vi "Get Class Functions C Description.vi"(8 "error in (no error)":errorcluster, 10 "Access Scope":T1(ring)=enum."public", 11 "LabVIEW Obj":refnum<class>) -> (0 "error out":errorcluster, 3 "Array":string[](array[string]))   [LabVIEW 2017]
uses:
  <userlib>/_OpenG.lib/string/string.llb/Trim Whitespace (String)__ogtk.vi
  <vilib>/Utility/VariantDataType/VariantType.lvlib
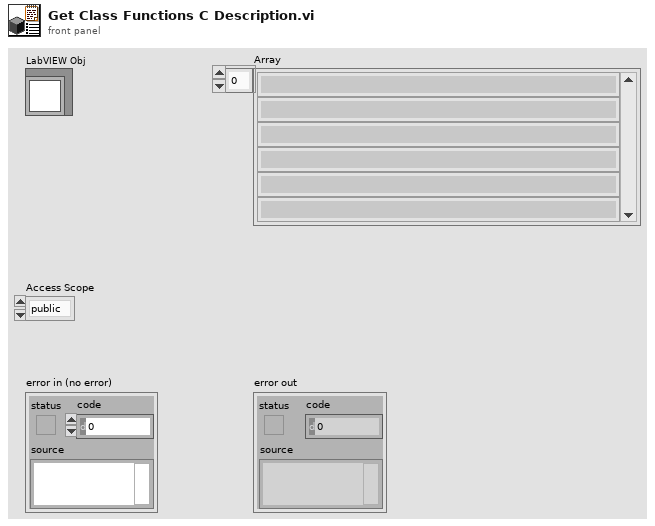
[diagram p1: front panel]
types:
  T1 = enum32{"invalid scope", "public", "private", "protected", "community"}
  T2 = typedef "VariantType.lvlib/VIInfo.ctl" = cluster{"Data1":i16, "Data2":i16, "Flags":u32[], "Modification Date":timestamp, "Asynchronous":bool, "NonFunctional":bool, "Subroutine":bool, "SubSystem":bool}
  T3 = typedef "Type Descriptor Enumeration__ogtk.ctl" = enum8{"<Null>", "I8", "I16", "I32", "I64", "U8", "U16", "U32", "U64", "SGL", "DBL", "EXT", "CSG", "CDB", "CXT", "0x0F", "0x10", "0x11", "0x12", "0x13", "0x14", "Enum U8", "Enum U16", "Enum U32", "Enum U64", "SGL PQ", "DBL PQ", "EXT PQ", "CSG PQ", "CDB PQ", "CXT PQ", "0x1F", "0x20", "Boolean", "0x22", "0x23", "0x24", "0x25", "0x26", "0x27", "0x28", "0x29", "0x2A", "0x2B", "0x2C", "0x2D", "0x2E", "0x2F", "String", "0x31", "Path", "Pict", "0x34", "0x35", "0x36", "DAQ", "0x38", "0x39", "0x3A", "0x3B", "0x3C", "0x3D", "0x3E", "0x3F", "Array", "0x41", "0x42", "0x43", "0x44", "0x45", "0x46", "0x47", "0x48", "0x49", "0x4A", "0x4B", "0x4C", "0x4D", "0x4E", "0x4F", "Cluster", "0x51", "0x52", "Variant", "Waveform", "0x55", "0x56", "0x57", "0x58", "0x59", "0x5A", "0x5B", "0x5C", "0x5D", "0x5E", "0x5F", "0x60", "0x61", "0x62", "0x63", "0x64", "0x65", "0x66", "0x67", "0x68", "0x69", "0x6A", "0x6B", "0x6C", "0x6D", "0x6E", "0x6F", "Refnum"}
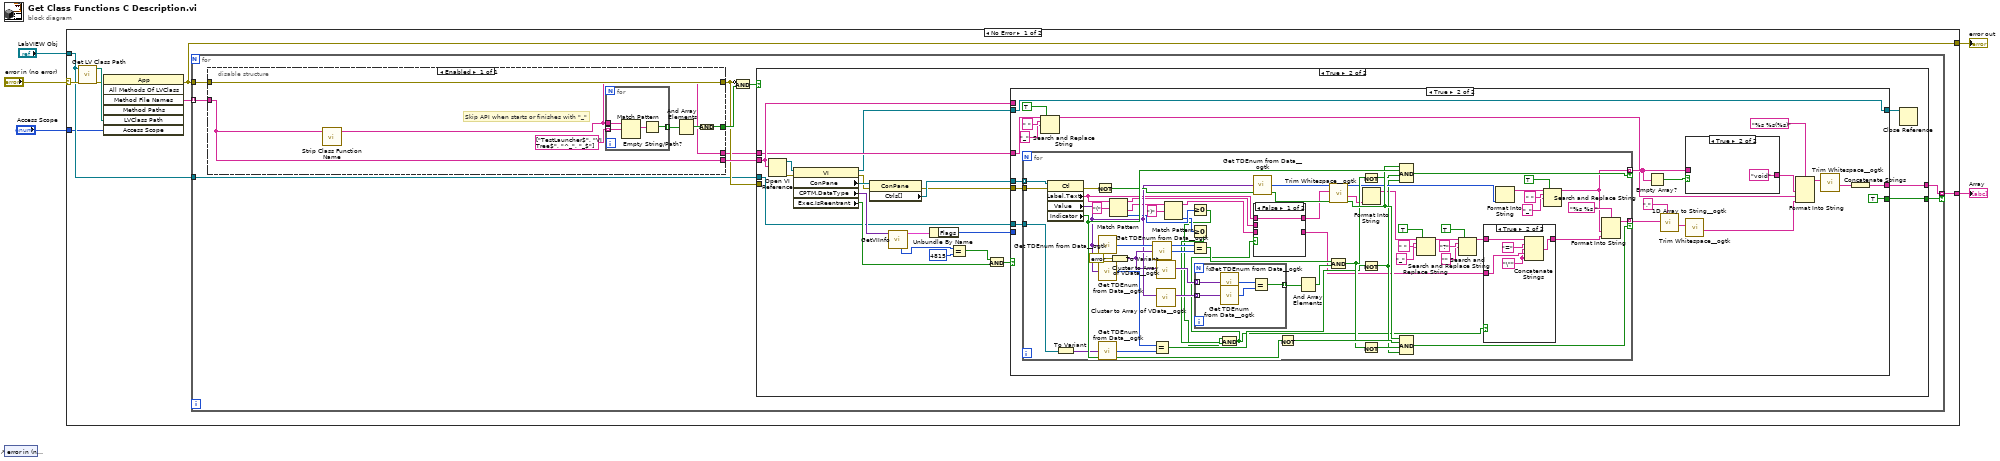
[diagram p0: block diagram]
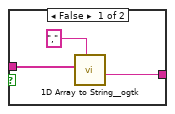
[diagram p4: hidden frame]
diagram:
  n1 = control-ref of="error in (no error)"() -> ()  [unwired: 1 out]
  n2 = case shown="No Error" "error in (no error)" {
    selector: "error in (no error)" -> [w12 w155]
    tunnel: [w9 w155] -> w4
    tunnel: "LabVIEW Obj" -> [w7 _]
    tunnel: [w8 _] -> w2
    tunnel: "Access Scope" -> [w6 _]
    frame No Error {
      n3 = call <vilib>:"Get LV Class Path.vi"("error in (no error)"=w12, "object"=w7) -> ("error out"=w10:errorcluster, "class path"=w13:path)  [unwired: 8 in]
      n4 = invoke class="App" method="All Methods Of LVClass"(error in=w10, "LVClass Path"=w13, "Access Scope"=w6) -> (error out=w9:errorcluster, "Method File Names"=w11:string[])  [unwired: 4 in, 5 out]
      n5 = for {
        tunnel: w11 -> [w19] mode=indexing
        tunnel: [w23] -> w8 mode=indexing if=w22
        tunnel: w9 -> [w20]
        tunnel: w7 -> [w14]
        n6 = disable-structure shown="Enabled" {
          disable-tunnel: [w24] -> w21
          disable-tunnel: w20 -> [w27]
          disable-tunnel: w19 -> [w24]
          disable-tunnel: [w26] -> w18
          disable-tunnel: [w27] -> w16
          disable-tunnel: [w25] -> w15
          frame Enabled {
            # "Skip API when starts or finishes with \"_\""
            n7 = call "Strip Class Function Name.vi"("File Full Path Name"=w24) -> ("Function Name"=w25:string)  [unwired: 2 in, 2 out]
            n8 = for {
              tunnel: w25 -> [w34]
              tunnel: string[] ["TestLauncher$", "VI Tree$", "^_", "_$"] -> [w33] mode=indexing
              tunnel: [w31] -> w28 mode=indexing
              n9 = Match Pattern(string=w34, regular expression=w33) -> (match substring=w32:string)  [unwired: 1 in, 3 out]
              n10 = Empty String/Path?(string/path=w32) -> (empty?=w31:bool)
            }
            n11 = And Array Elements(Boolean array=w28) -> (logical AND=w30:bool)
            n12 = Compound Arithmetic op=AND(w30) -> (w26:bool)
          }
        }
        n13 = Compound Arithmetic op=AND(invert w16, w18) -> (w17:bool)
        n14 = case shown="True" w17 {
          tunnel: [_ w55] -> w23
          tunnel: [_ w54] -> w22
          tunnel: w21 -> [_ w53]
          tunnel: w16 -> [_ _]
          tunnel: w15 -> [_ w52]
          tunnel: w14 -> [_ w35]
          frame False {
          }
          frame True {
            n15 = Open VI Reference(vi path=w53) -> (vi reference=w47:refnum<vi>, error out=w48:errorcluster)  [unwired: 5 in]
            n16 = property class="VI"(reference=w47, error in=w48) -> (reference out=w38:refnum<vi>, error out=w46:errorcluster, "ConPane"=w51:refnum<vi>, "CPTM.DataType"=w45:variant, "Exec.IsReentrant"=w39:bool)
            n17 = property class="ConPane"(reference=w51, error in=w46) -> (error out=w36:errorcluster, "Ctrls[]"=w50:refnum<vi>[])  [unwired: 1 out]
            n18 = call <vilib>:"GetVIInfo.vi"("Variant"=w45) -> ("VI Info"=w43:T2, "pattern"=w44:i16)  [unwired: 6 in, 3 out]
            n19 = Unbundle By Name(w43) -> ("Flags"=w42:u32[])
            n20 = Equal?(x=w44, y=i16 4815) -> (x = y?=w41:bool)
            n21 = Compound Arithmetic op=AND(w41, w39) -> (w40:bool)
            n22 = case shown="True" w40 {
              tunnel: [_ w57] -> w55
              tunnel: w50 -> [_ w76]
              tunnel: [_ TRUE] -> w54
              tunnel: w53 -> [_ _]
              tunnel: w52 -> [_ w61]
              tunnel: w42 -> [_ _]
              tunnel: w38 -> [w56 w77]
              tunnel: [w56 w77] -> w37
              tunnel: w36 -> [_ w69]
              tunnel: w35 -> [_ w67]
              frame False {
              }
              frame True {
                n23 = for {
                  tunnel: w76 -> [w140] mode=indexing
                  tunnel: [w102] -> w66 mode=indexing if=w133
                  tunnel: [w138] -> w74 mode=indexing if=w132
                  tunnel: w69 -> [w135]
                  tunnel: w67 -> [w116]
                  n24 = property class="Ctl"(reference=w140, error in=w135) -> (error out=w134:errorcluster, "Label.Text"=w95:string, "Value"=w115:variant, "Indicator"=w137:bool)  [unwired: 1 out]
                  n25 = To Variant(anything=w116) -> (Variant=w117:variant)
                  n26 = Not(x=w134) -> (.not. x?=w131:bool)
                  n27 = call <userlib>:"Get TDEnum from Data__ogtk.vi"("Data"=w115) -> ("Type Descriptor Enumeration"=w129:T3)  [unwired: 4 in]
                  n28 = call <userlib>:"Get TDEnum from Data__ogtk.vi"("Data"=w115) -> ("Type Descriptor Enumeration"=w114:T3)  [unwired: 4 in]
                  n29 = call <userlib>:"Get TDEnum from Data__ogtk.vi"("Data"=w117) -> ("Type Descriptor Enumeration"=w113:T3)  [unwired: 4 in]
                  n30 = Match Pattern(string=w95, regular expression="(") -> (before substring=w93:string, after substring=w88:string, offset past match=w99:i32)  [unwired: 1 in, 1 out]
                  n31 = To Variant(anything=errorcluster {"status"=FALSE, "code"=0, "source"=""} ("error in (no error)")) -> (Variant=w127:variant)
                  n32 = call <userlib>:"Get TDEnum from Data__ogtk.vi"("Data"=w127) -> ("Type Descriptor Enumeration"=w128:T3)  [unwired: 4 in]
                  n33 = Equal?(x=w114, y=w113) -> (x = y?=w112:bool)
                  n34 = call <userlib>:"Cluster to Array of VData__ogtk.vi"("Cluster"=w127) -> ("Array of VData"=w126:variant[])  [unwired: 9 in, 1 out]
                  n35 = call <userlib>:"Cluster to Array of VData__ogtk.vi"("Cluster"=w115) -> ("Array of VData"=w125:variant[])  [unwired: 9 in, 1 out]
                  n36 = Match Pattern(string=w88, regular expression=")") -> (before substring=w89:string, offset past match=w98:i32)  [unwired: 1 in, 2 out]
                  n37 = Greater Or Equal To 0?(x=w99) -> (x >= 0?=w96:bool)
                  n38 = Greater Or Equal To 0?(x=w98) -> (x >= 0?=w97:bool)
                  n39 = Equal?(x=w129, y=w128) -> (x = y?=w124:bool)
                  n40 = for {
                    tunnel: w126 -> [w154] mode=indexing
                    tunnel: w125 -> [w153] mode=indexing
                    tunnel: [w150] -> w123 mode=indexing
                    n41 = call <userlib>:"Get TDEnum from Data__ogtk.vi"("Data"=w154) -> ("Type Descriptor Enumeration"=w152:T3)  [unwired: 4 in]
                    n42 = call <userlib>:"Get TDEnum from Data__ogtk.vi"("Data"=w153) -> ("Type Descriptor Enumeration"=w151:T3)  [unwired: 4 in]
                    n43 = Equal?(x=w152, y=w151) -> (x = y?=w150:bool)
                  }
                  n44 = And(x=w96, y=w97) -> (x .and. y?=w92:bool)
                  n45 = call <userlib>:"Get TDEnum from Data__ogtk.vi"("Data"=w115) -> ("Type Descriptor Enumeration"=w118:T3)  [unwired: 4 in]
                  n46 = case shown="False" w92 {
                    tunnel: [w147 w149] -> w94
                    tunnel: w95 -> [w147 _]
                    tunnel: w93 -> [_ w149]
                    tunnel: [_ w148] -> w90
                    tunnel: w89 -> [_ w148]
                    frame False {
                    }
                    frame True {
                    }
                  }
                  n47 = Not(x=w137) -> (.not. x?=w136:bool)
                  n48 = And Array Elements(Boolean array=w123) -> (logical AND=w121:bool)
                  n49 = call-poly <userlib>:"Trim Whitespace__ogtk.vi"("String in"=w94) -> ("String out"=w87:string)  [unwired: 6 in]
                  n50 = Compound Arithmetic op=AND(w124, w121) -> (w122:bool)
                  n51 = Not(x=w122) -> (.not. x?=w119:bool)
                  n52 = Not(x=w122) -> (.not. x?=w120:bool)
                  n53 = Format Into String(w87) -> (resulting string=w103:string)  [unwired: 3 in, 1 out]
                  n54 = Not(x=w112) -> (.not. x?=w111:bool)
                  n55 = Compound Arithmetic op=AND(w131, w137, w119, w111) -> (w133:bool)
                  n56 = Compound Arithmetic op=AND(w131, w136, w120, w111) -> (w132:bool)
                  n57 = Search and Replace String(replace all?=TRUE ("replace all? (F)"), input string=w103, search string=" ", replace string="_" ("replace string (\"\")")) -> (result string=w83:string)  [unwired: 4 in, 3 out]
                  n58 = Search and Replace String(replace all?=TRUE ("replace all? (F)"), input string=w83, search string="?", replace string="" ("replace string (\"\")")) -> (result string=w82:string)  [unwired: 4 in, 3 out]
                  n59 = case shown="True" w92 {
                    tunnel: w82 -> [w141 w145]
                    tunnel: [w141 w146] -> w91
                    tunnel: w90 -> [_ w143]
                    frame False {
                    }
                    frame True {
                      w142 = "\"" ("string")
                      n60 = Concatenate Strings(w145, "=" ("string"), w142, w143, w142) -> (w146:string)
                    }
                  }
                  n61 = Format Into String(w118) -> (resulting string=w110:string)  [unwired: 3 in, 1 out]
                  n62 = Search and Replace String(replace all?=TRUE ("replace all? (F)"), input string=w110, search string=" ", replace string="_" ("replace string (\"\")")) -> (result string=w102:string)  [unwired: 4 in, 3 out]
                  n63 = Format Into String(format string="%s %s ", w102, w91) -> (resulting string=w138:string)  [unwired: 2 in, 1 out]
                }
                n64 = Search and Replace String(replace all?=TRUE ("replace all? (F)"), input string=w61, search string=" ", replace string="_" ("replace string (\"\")")) -> (result string=w60:string)  [unwired: 4 in, 3 out]
                n65 = Empty Array?(array=w66) -> (empty?=w65:bool)
                n66 = call <userlib>:"1D Array to String__ogtk.vi"("delimiter (Tab)"=",", "Array of Strings"=w74) -> ("delimited string"=w71:string)  [unwired: 9 in]
                n67 = case shown="True" w65 {
                  tunnel: [w79 "void" ("delimited string")] -> w72
                  tunnel: w66 -> [w78 _]
                  frame False {
                    n68 = call <userlib>:"1D Array to String__ogtk.vi"("delimiter (Tab)"=",", "Array of Strings"=w78) -> ("delimited string"=w79:string)  [unwired: 9 in]
                  }
                  frame True {
                  }
                }
                n69 = call-poly <userlib>:"Trim Whitespace__ogtk.vi"("String in"=w71) -> ("String out"=w58:string)  [unwired: 6 in]
                n70 = Format Into String(format string="%s %s(%s)", w72, w60, w58) -> (resulting string=w70:string)  [unwired: 2 in, 1 out]
                n71 = call-poly <userlib>:"Trim Whitespace__ogtk.vi"("String in"=w70) -> ("String out"=w59:string)  [unwired: 6 in]
                n72 = Concatenate Strings(w59) -> (w57:string)
              }
            }
            n73 = Close Reference(reference=w37) -> ()  [unwired: 1 in, 1 out]
          }
        }
      }
    }
    frame Error {
    }
  }
  "error out" <- w4
  "Array" <- w2
